vi "Test Virtual Thermometer from CSV with Alarming.vi"(11 "Test Case In":refnum<class "Test Instrument Manager.lvclass">) -> (0 "error out":errorcluster, 3 "Test Case Out":refnum<class "Test Instrument Manager.lvclass">)   [LabVIEW 2024, in "Test Instrument Manager.lvclass"]
uses:
  Test Instrument Manager.lvclass
  Test Instrument Manager.lvclass/Test Instrument Manager.ctl
  Alarming-Actor/Source/Alarming Actor UI/Alarming Actor UI.lvclass
  Alarming-Actor/Source/Alarming Actor/Alarming Actor/Alarming Actor.lvclass
  Source/Alarming Strategy/Alarming Actor Strategy.lvclass
  Source/Instrument Manager/Instrument Manager.lvclass
  Source/Interfaces/IRead Temperature/IRead Temperature.lvclass
  Source/Interfaces/IVirtual Instrument/IVirtual Instrument.lvclass
  <vilib>/Astemes/LUnit/Test Case.lvclass
  cceb4bd8-3600-4d38-a702-34d5b4246d90.vi
  Alarming-Actor/Source/Alarming Actor/Alarming Actor/Alarming Level.ctl
panel:
  out "Time Stamp":timestamp format="%<%x %.3X>T"
  out "Waveform Chart":dbl(graph)
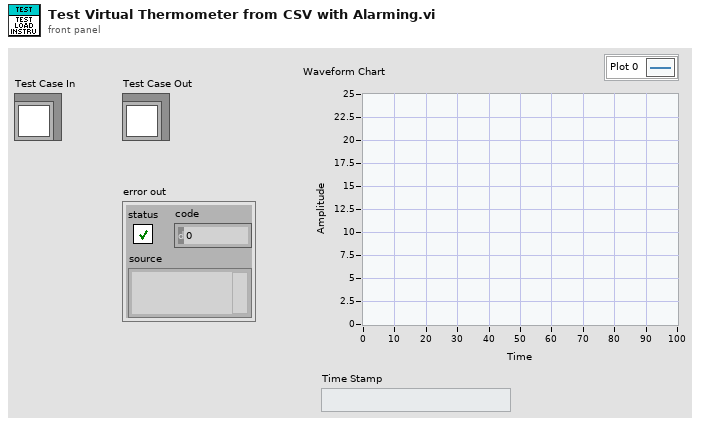
[diagram p1: front panel]
types:
  T1 = typedef "Alarming Actor.lvlib/Alarming Actor.lvclass/Alarming Level.ctl" = enum16{"Unknown", "OK", "Warning", "Critical"}
  T2 = cluster{"Identifier":string, "Alarming Level":T1}
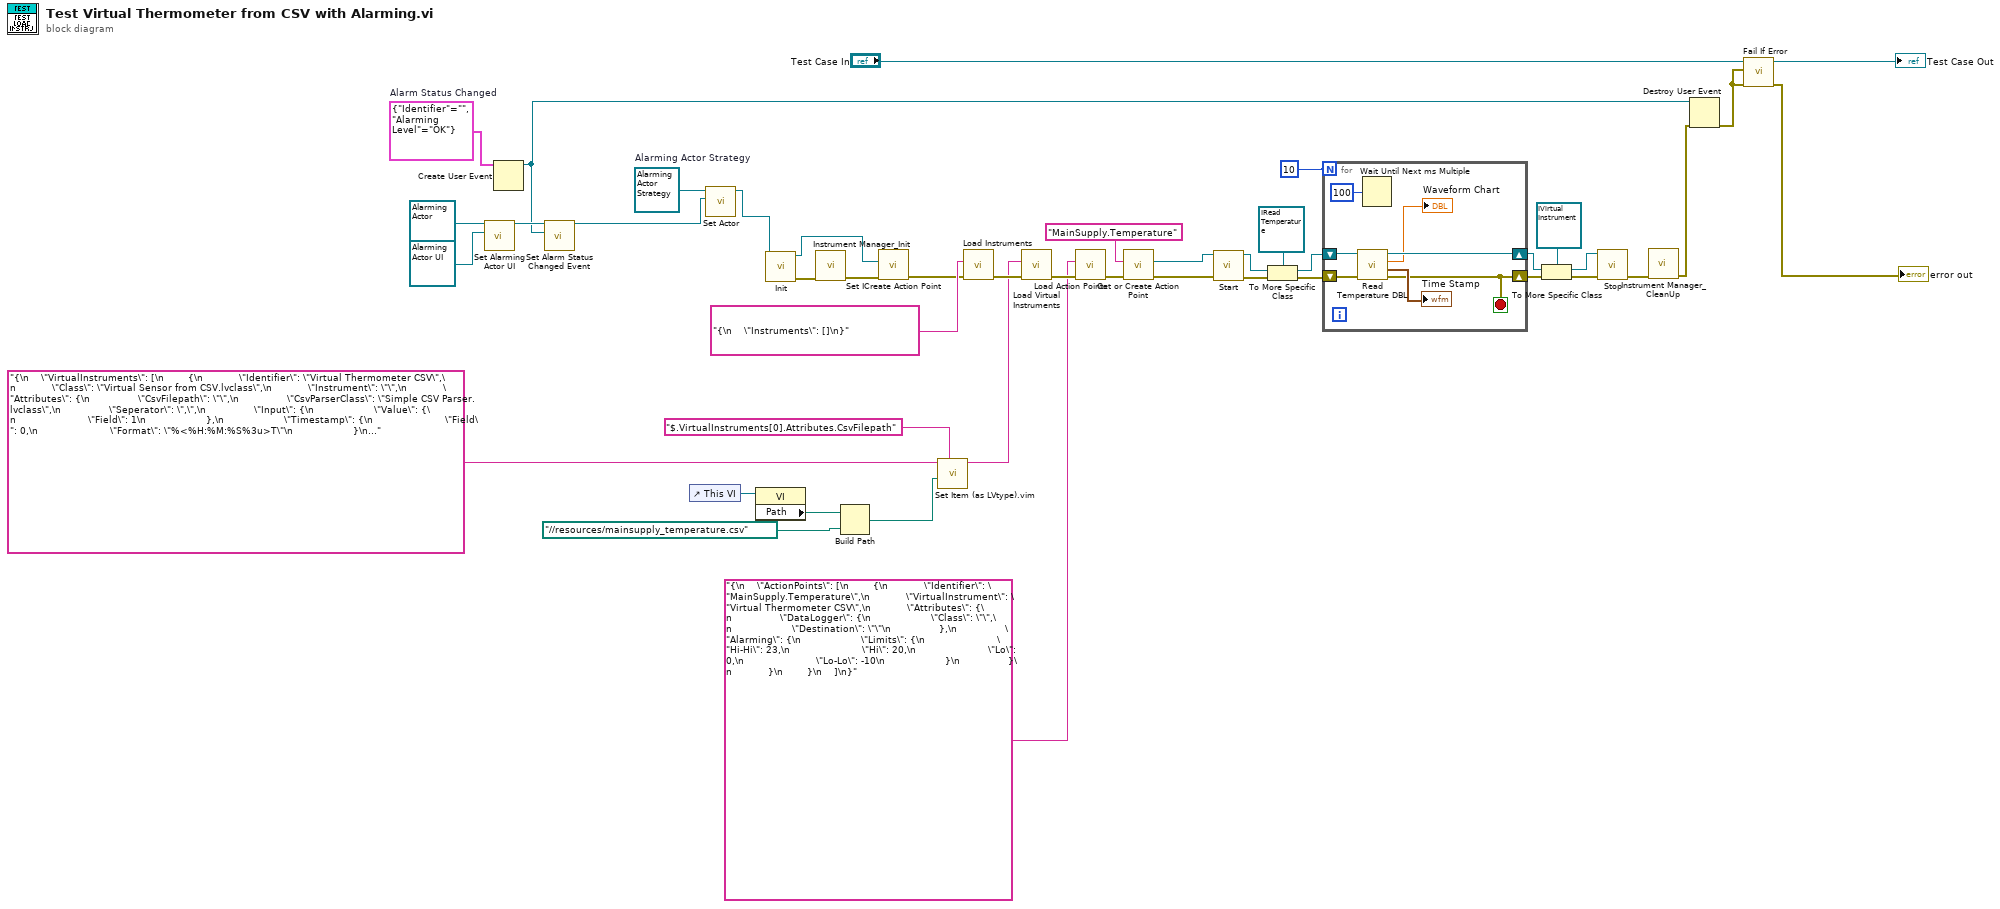
[diagram p0: block diagram]
diagram:
  w7 = T2 {"Identifier"="", "Alarming Level"=enum."OK"}  # Alarm Status Changed
  w14 = refnum<class "Alarming Actor Strategy.lvclass"> refnum  # Alarming Actor Strategy
  n1 = call "Set Alarming Actor UI.vi"("UI Actor"=refnum<class "Alarming Actor UI.lvclass"> refnum ("Alarming Actor UI.lvlib:Alarming Actor UI.lvclass"), "Alarming Actor in"=refnum<class "Alarming Actor.lvclass"> refnum ("Alarming Actor.lvlib:Alarming Actor.lvclass")) -> ("Alarming Actor out"=w9:refnum<class "Alarming Actor.lvclass">)  [unwired: 9 in]
  n2 = Create User Event(user event datatype=w7) -> (user event=w3:refnum<user-event>)  [unwired: 1 in, 1 out]
  n3 = call "Set Alarm Status Changed Event.vi"("Alarm Status Changed"=w3, "Alarming Actor in"=w9) -> ("Alarming Actor out"=w6:refnum<class "Alarming Actor.lvclass">)  [unwired: 9 in]
  n4 = control-ref of="This VI"() -> (w19:refnum<vi>)
  n5 = call-dynamic "Set Actor.vi"("Actor"=w6, "Alarming Strategy in"=w14) -> ("Alarming Strategy out"=w11:refnum<class "Alarming Actor Strategy.lvclass">)  [unwired: 9 in]
  n6 = property class="VI"(reference=w19) -> ("Path"=w18:path)  [unwired: 1 in, 2 out]
  n7 = call-dynamic "Init.vi"("Alarming Strategy in"=w11) -> ("error out"=w5:errorcluster, "Alarming Strategy out"=w12:refnum<class "Alarming Actor Strategy.lvclass">)  [unwired: 9 in]
  n8 = call "Instrument Manager_Init.vi"("Error In"=w5) -> ("Error Out"=w4:errorcluster)  [unwired: 9 in, 1 out]
  n9 = Build Path(base path=w18, name or relative path=path "../../resources/mainsupply_temperature.csv") -> (appended path=w16:path)
  n10 = call "Set ICreate Action Point.vi"("Error In"=w4, "ICreate Action Point"=w12) -> ("Error Out"=w13:errorcluster)  [unwired: 9 in]
  n11 = call "Set Item (as LVtype).vim"("$Path or Item Name"="$.VirtualInstruments[0].Attributes.CsvFilepath", "Anything"=w16, "JSON"="{\n    \"VirtualInstruments\": [\n        {\n            \"Identifier\": \"Virtual Thermometer CSV\",\n            \"Class\": \"Virtual Sensor from CSV.lvclass\",\n            \"Instrument\": \"\",\n            \"Attributes\": {\n                \"CsvFilepath\": \"\",\n                \"CsvParserClass\": \"Simple CSV Parser.lvclass\",\n                \"Seperator\": \",\",\n                \"Input\": {\n                    \"Value\": {\n                        \"Field\": 1\n                    },\n                    \"Timestamp\": {\n                        \"Field\": 0,\n                        \"Format\": \"%<%H:%M:%S%3u>T\"\n                    }\n                }\n            }\n        }\n    ]\n}") -> ("<JSON>"=w20:string)  [unwired: 5 in, 2 out]
  n12 = call "Load Instruments.vi"("Error In"=w13, "Source"="{\n    \"Instruments\": []\n}") -> ("Error Out"=w42:errorcluster)  [unwired: 9 in]
  n13 = call "Load Virtual Instruments.vi"("Error In"=w42, "Source"=w20) -> ("Error Out"=w39:errorcluster)  [unwired: 9 in]
  n14 = call "Load Action Points.vi"("Error In"=w39, "Source"="{\n    \"ActionPoints\": [\n        {\n            \"Identifier\": \"MainSupply.Temperature\",\n            \"VirtualInstrument\": \"Virtual Thermometer CSV\",\n            \"Attributes\": {\n                \"DataLogger\": {\n                    \"Class\": \"\",\n                    \"Destination\": \"\"\n                },\n                \"Alarming\": {\n                    \"Limits\": {\n                        \"Hi-Hi\": 23,\n                        \"Hi\": 20,\n                        \"Lo\": 0,\n                        \"Lo-Lo\": -10\n                    }\n                }\n            }\n        }\n    ]\n}") -> ("Error Out"=w37:errorcluster)  [unwired: 9 in]
  n15 = call "Get or Create Action Point.vi"("Error In"=w37, "Action Point Identifier"="MainSupply.Temperature") -> ("Error Out"=w34:errorcluster, "IAction Point"=w33:refnum<class "IVirtual Instrument.lvclass">)  [unwired: 8 in]
  n16 = call-dynamic "Start.vi"("error in"=w34, "IRunnable in"=w33) -> ("error out"=w32:errorcluster, "IRunnable out"=w29:refnum<class "IVirtual Instrument.lvclass">)  [unwired: 8 in]
  n17 = To More Specific Class(target class=refnum<class "IRead Temperature.lvclass"> refnum ("IRead Temperature.lvclass"), reference=w29, error in=w32) -> (specific class reference=w27:refnum<class "IRead Temperature.lvclass">, error out=w30:errorcluster)
  n18 = for {
    N: 10 -> [_]
    shift-right: [w45] -> w35
    shift-left: w30 -> [w51]
    shift-right: [w49] -> w25
    shift-left: w27 -> [w50]
    stop <- w45 stop-if-true
    n19 = call-dynamic "Read Temperature DBL.vi"("error in"=w51, "IRead Temperature in"=w50) -> ("error out"=w45:errorcluster, "Time Stamp"=→"Time Stamp":timestamp, "Temperature"=→"Waveform Chart":dbl, "IRead Temperature out"=w49:refnum<class "IRead Temperature.lvclass">)  [unwired: 6 in]
    n20 = Wait Until Next ms Multiple(millisecond multiple=u32 100) -> ()  [unwired: 1 out]
  }
  n21 = To More Specific Class(target class=refnum<class "IVirtual Instrument.lvclass"> refnum ("IVirtual Instrument.lvclass"), reference=w25, error in=w35) -> (specific class reference=w24:refnum<class "IVirtual Instrument.lvclass">, error out=w26:errorcluster)
  n22 = call-dynamic "Stop.vi"("error in"=w26, "IRunnable in"=w24) -> ("error out"=w31:errorcluster)  [unwired: 8 in, 1 out]
  n23 = call "Instrument Manager_CleanUp.vi"("Error In"=w31) -> ("Error Out"=w2:errorcluster)  [unwired: 10 in]
  n24 = Destroy User Event(user event=w3, error in=w2) -> (error out=w1:errorcluster)
  n25 = call <vilib>:"Fail If Error.vi"("error in (no error)"=w1, "Assert error"=w1, "LUnit Test Case In"="Test Case In") -> ("error out"=→"error out":errorcluster, "LUnit Test Case Out"=→"Test Case Out":refnum<class "Test Instrument Manager.lvclass">)  [unwired: 7 in]
